vi "初始化流程 文件-连接-结构-设备.vi"(8 "错误输出":errorcluster) -> (0 "error out":errorcluster, 3 "探测器信息[]":T1[](array[typedef]))   [LabVIEW 2017]
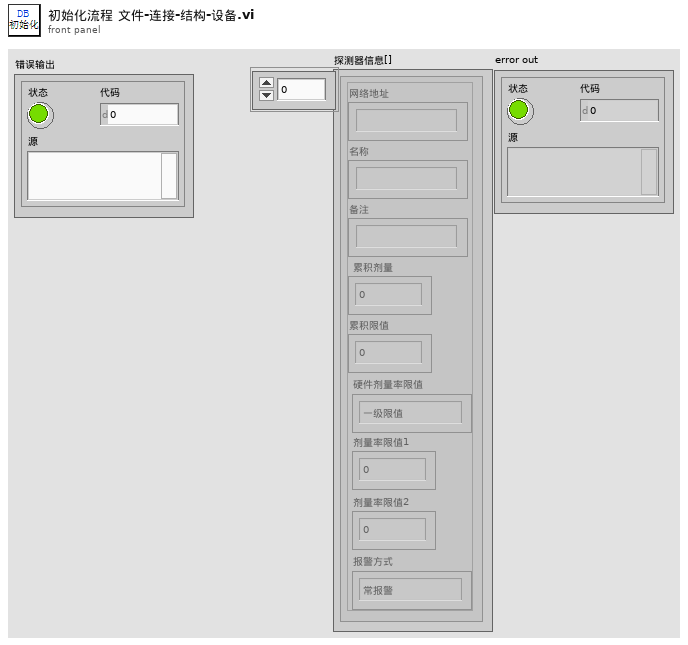
[diagram p1: front panel]
types:
  T1 = typedef "探测器信息.ctl" = cluster{"网络地址":string, "名称":string, "备注":string, "累积剂量":dbl, "累积限值":dbl, "硬件剂量率限值":T2, "剂量率限值1":dbl, "剂量率限值2":dbl, "报警方式":T3}
  T2 = typedef "探头剂量率限值选择.ctl" = enum16{"一级限值", "二级限值"}
  T3 = typedef "报警方式选择.ctl" = enum16{"常报警", "自动静音", "手动静音"}
  T4 = typedef "DB动作类型.ctl" = enum16{"DB-文件初始化+连接", "DB-断开连接", "DB-结构初始化", "DB-加载设备", "DB-检查连接状态", "设备-登记新设备+数据表", "设备-删除设备", "设备-修改网址", "设备-修改名称+转移数据", "设备-修改备注", "设备-修改限值", "设备-累积校准", "设备-重排", "数据-获取全部", "数据-删除数据", "数据-写改累积记录+改累积剂量", "读变量-全部设备"}
  T5 = typedef "DB动作与数据.ctl" = cluster{"动作类型":T4, "输入数据":variant}
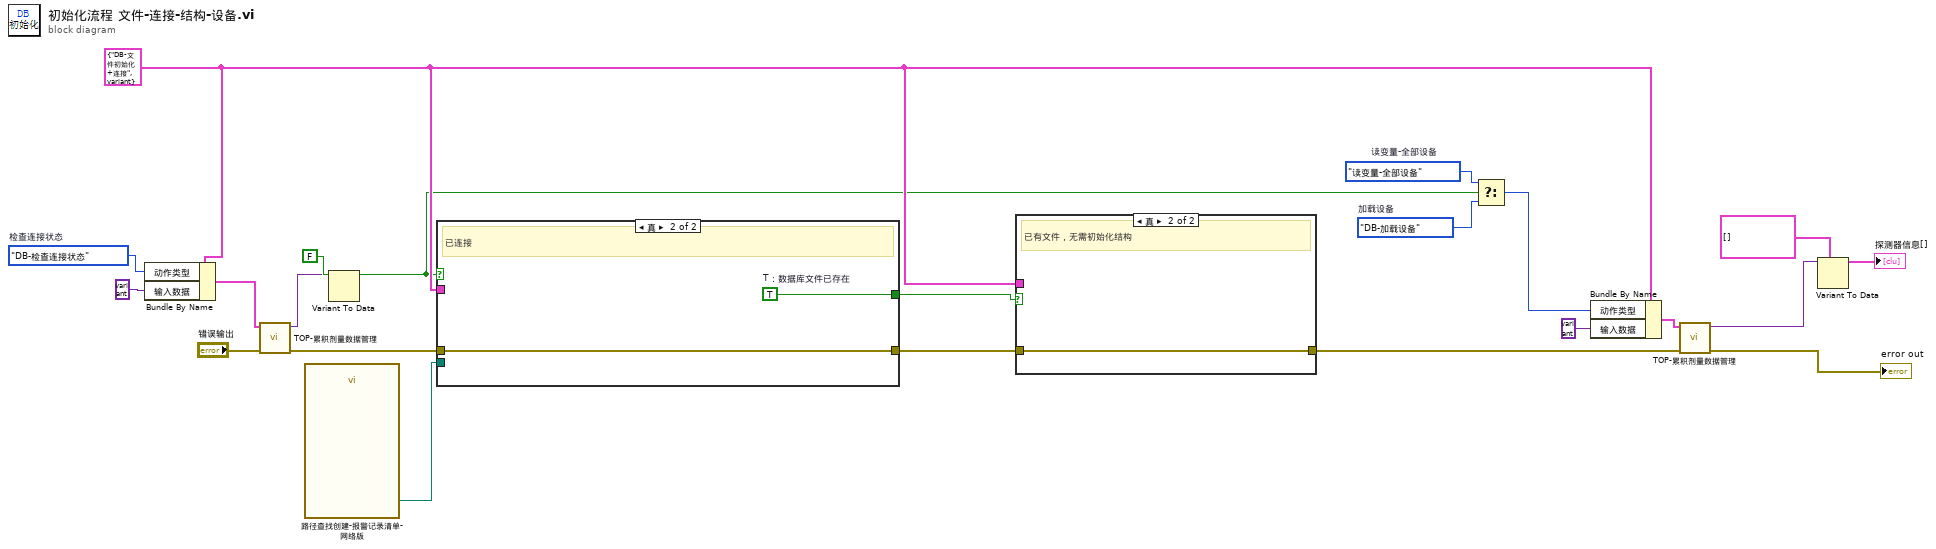
[diagram p0: block diagram]
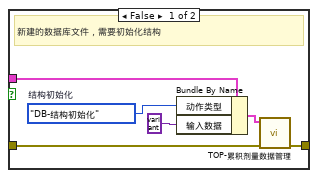
[diagram p2: hidden frame]
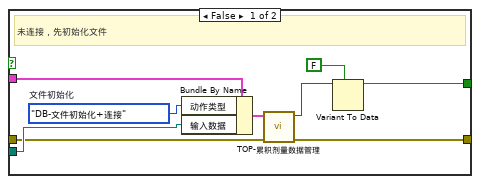
[diagram p3: hidden frame]
diagram:
  w2 = DB动作类型."读变量-全部设备"  # 读变量-全部设备
  w3 = DB动作类型."DB-加载设备"  # 加载设备
  w18 = DB动作类型."DB-检查连接状态"  # 检查连接状态
  w14 = T5 {"动作类型"=enum."DB-文件初始化+连接", "输入数据"=variant} ("DB动作集")
  n1 = Bundle By Name(cluster=w14, "动作类型"=w18, "输入数据"=variant) -> (w20:T5)
  n2 = call "TOP-累积剂量数据管理.vi"("错误输出"="错误输出", "DB动作集"=w20) -> ("error out"=w13:errorcluster, "输出数据"=w21:variant)  [unwired: 8 in]
  n3 = call "路径查找创建-报警记录清单-网络版.vi"() -> ("累积剂量数据库"=w17:path)  [unwired: 2 in, 13 out]
  n4 = Variant To Data(type=FALSE, Variant=w21) -> (data=w4:bool)  [unwired: 1 in, 1 out]
  n5 = case shown="真" w4 {
    tunnel: w14 -> [w29 _]
    tunnel: w17 -> [w28 _]
    tunnel: [w25 w33] -> w15
    tunnel: w13 -> [w24 w32]
    tunnel: [w23 w32] -> w12
    frame False {
      w31 = DB动作类型."DB-文件初始化+连接"  # 文件初始化
      # "未连接，先初始化文件"
      n6 = Bundle By Name(cluster=w29, "动作类型"=w31, "输入数据"=w28) -> (w30:T5)
      n7 = call "TOP-累积剂量数据管理.vi"("错误输出"=w24, "DB动作集"=w30) -> ("error out"=w23:errorcluster, "输出数据"=w26:variant)  [unwired: 8 in]
      n8 = Variant To Data(type=FALSE, Variant=w26) -> (data=w25:bool)  [unwired: 1 in, 1 out]
    }
    frame True {
      w33 = TRUE  # T：数据库文件已存在
      # "已连接"
    }
  }
  n9 = case shown="真" w15 {
    tunnel: [w39 w40] -> w16
    tunnel: w14 -> [w36 _]
    tunnel: w12 -> [w35 w40]
    frame False {
      w37 = DB动作类型."DB-结构初始化"  # 结构初始化
      # "新建的数据库文件，需要初始化结构"
      n10 = Bundle By Name(cluster=w36, "动作类型"=w37, "输入数据"=variant) -> (w38:T5)
      n11 = call "TOP-累积剂量数据管理.vi"("错误输出"=w35, "DB动作集"=w38) -> ("error out"=w39:errorcluster)  [unwired: 8 in, 1 out]
    }
    frame True {
      # "已有文件，无需初始化结构"
    }
  }
  n12 = Select(t=w2, s=w4, f=w3) -> (s? t:f=w1:T4)
  n13 = Bundle By Name(cluster=w14, "动作类型"=w1, "输入数据"=variant) -> (w11:T5)
  n14 = call "TOP-累积剂量数据管理.vi"("错误输出"=w16, "DB动作集"=w11) -> ("error out"=→"error out":errorcluster, "输出数据"=w9:variant)  [unwired: 8 in]
  n15 = Variant To Data(type=T1[] [] ("探测器清单"), Variant=w9) -> (data=→"探测器信息[]":T1[])  [unwired: 1 in, 1 out]
